vi "ARM_GLOBALS.vi"() -> ()   [LabVIEW 2023]
uses:
  <vilib>/Rock Robotics/WPI/ThirdParty/JAS_Junk/TrajLib/Enum/DCMOTOR_TYPES_ENUM.ctl
  <vilib>/Rock Robotics/WPI/ThirdParty/JAS_Junk/TrajLib/Trajectory_Library.lvlib
panel:
  out "Filtered_ArmSpeed_RadPerSec":dbl
  out "Filtered_ArmAngle_Deg":dbl
  out "FeedForward On?":bool
  out "ArmSpeed_RadPerSec":dbl
  out "ArmAngle_Deg":dbl
  out "Base Motor params":cluster{"Motor Type":T1, "Gear Ratio":dbl}
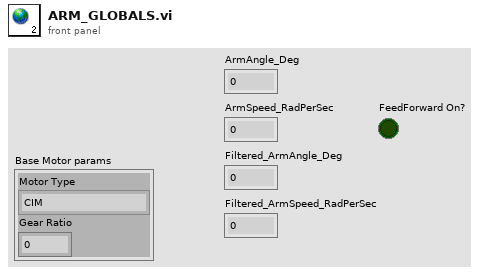
[diagram p1: front panel]
types:
  T1 = typedef "Trajectory_Library.lvlib/DCMOTOR_TYPES_ENUM.ctl" = enum16{"CIM", "AndyMark 9015", "Andy Mark RS 775 125", "Bag", "BaneBots RS 550", "BaneBots RS 775", "Falcon 500", "Mini CIM", "NEO", "NEO 550", "Romi BuiltIn", "Vex 775 Pro", "Snow Blower AM 2235A", "Bosch Seat AM 3493"}
diagram:
